vi "Flatten Value.vi"(8 "error in (no error)":errorcluster, 11 "Boolean in":refnum<class "Test Executive.lvclass">) -> (0 "error out":errorcluster, 2 "Value":string, 3 "Boolean out":refnum<class "Test Executive.lvclass">)   [LabVIEW 2017, in "Custom Type Test Executive.lvlib" / "Test Executive.lvclass"]
uses:
  <vilib>/gpm_packages/@cs/test-executive/Source/Custom Type Test Executive/Test Executive Data Type/Test Executive.lvclass
  <vilib>/gpm_packages/@cs/test-executive/Source/Custom Type Test Executive/Test Executive Data Type/Test Executive.lvclass/Test Executive.ctl
  <vilib>/gpm_packages/@cs/test-executive/Source/Test Executive/ITestExecutive/ITest Executive.lvclass
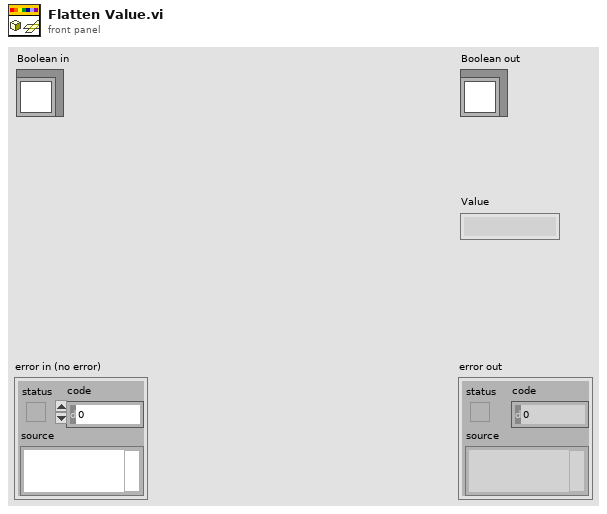
[diagram p1: front panel]
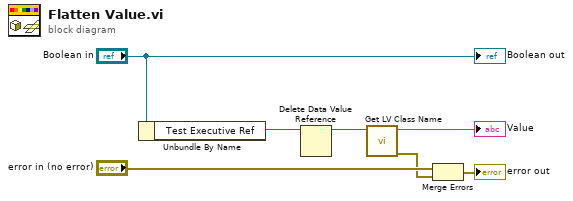
[diagram p0: block diagram]
diagram:
  n1 = Unbundle By Name("Boolean in") -> ("Test Executive Ref"=w4:refnum<data-value>)
  n2 = Delete Data Value Reference(data value reference=w4) -> (data value=w3:refnum<class "ITest Executive.lvclass">)  [unwired: 1 in, 1 out]
  n3 = call <vilib>:"Get LV Class Name.vi"("object"=w3) -> ("error out"=w2:errorcluster, "class name"=→"Value":string)  [unwired: 9 in]
  n4 = Merge Errors("error in (no error)", w2) -> (→"error out":errorcluster)
  "Boolean out" <- "Boolean in"
